vi "Czasomierz FVG.vi"(7 "Akcja":enum16{"Reset", "Wait"}(ring), 10 "Czas (s)":dbl) -> (2 "Elapsed?":bool)   [LabVIEW 2013]
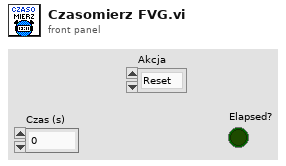
[diagram p1: front panel]
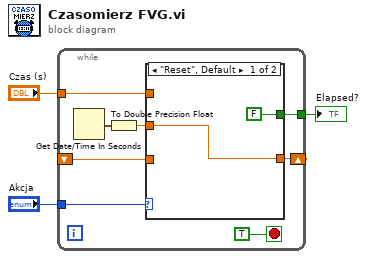
[diagram p0: block diagram]
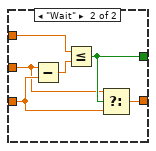
[diagram p2: hidden frame]
diagram:
  n1 = while {
    tunnel: "Akcja" -> [w11]
    shift-right: [w7] -> _
    shift-left: _ -> [w6]
    tunnel: "Czas (s)" -> [w5]
    tunnel: [w4] -> w1
    stop <- TRUE stop-if-true
    n2 = Get Date/Time In Seconds() -> (seconds since 1Jan1904=w9:timestamp)
    n3 = To Double Precision Float(number=w9) -> (double precision float=w8:dbl)
    n4 = case shown="\"Reset\", Default" w11 {
      tunnel: w8 -> [w13 w14]
      tunnel: [w13 w15] -> w7
      tunnel: w6 -> [_ w16]
      tunnel: w5 -> [_ w18]
      tunnel: [FALSE w17] -> w4
      frame "Reset", Default {
      }
      frame "Wait" {
        n5 = Subtract(x=w14, y=w16) -> (x-y=w19:dbl)
        n6 = Less Or Equal?(x=w18, y=w19) -> (x <= y?=w17:bool)
        n7 = Select(t=w14, s=w17, f=w16) -> (s? t:f=w15:dbl)
      }
    }
  }
  "Elapsed?" <- w1
